vi "Bang-bang.vi"(1 "Feedback":dbl, 2 "Target":dbl, 3 "Tolerance":dbl, 4 "Slow point":dbl, 5 "Low Speed":dbl, 6 "High Speed":dbl) -> (0 "Out speed":dbl)   [LabVIEW 2015]
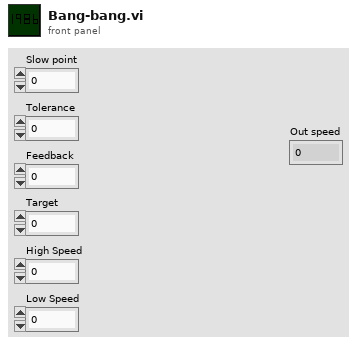
[diagram p1: front panel]
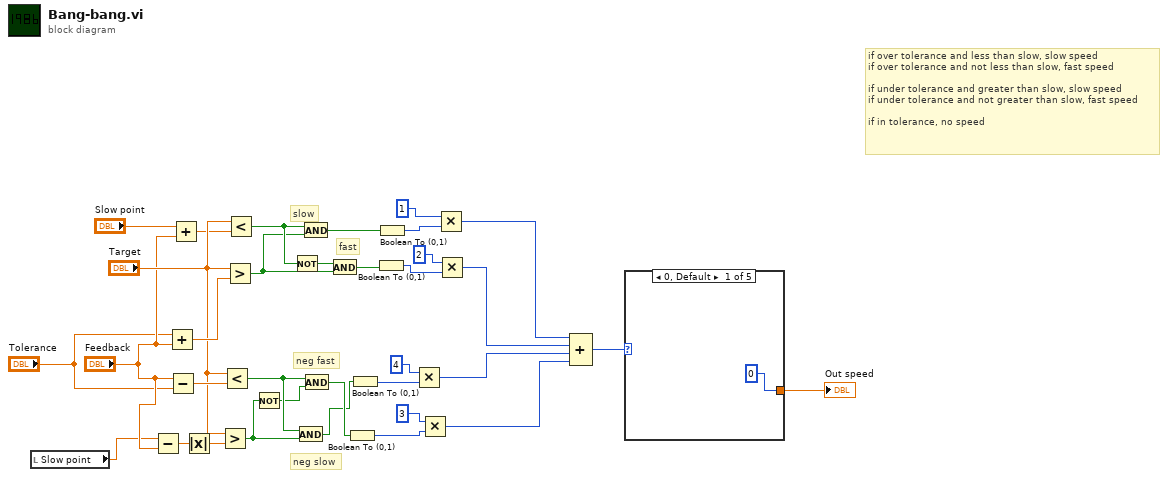
[diagram p0: block diagram]
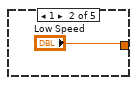
[diagram p2: hidden frame]
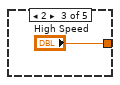
[diagram p3: hidden frame]
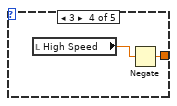
[diagram p4: hidden frame]
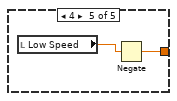
[diagram p5: hidden frame]
diagram:
  # "fast"
  # "neg fast"
  # "neg slow"
  # "slow"
  # "if over tolerance and less than slow, slow speed\nif over tolerance and not less than slow, fast speed\n\nif under tolerance and greater than slow, slow speed\nif under tolerance and not greater than slow, fast speed\n\nif in tolerance, no speed"
  n1 = local read "Slow point"() -> (w28:dbl)
  n2 = Subtract(x=w28, y="Feedback") -> (x-y=w2:dbl)
  n3 = Add(x="Tolerance", y="Feedback") -> (x+y=w34:dbl)
  n4 = Subtract(x="Feedback", y="Tolerance") -> (x-y=w33:dbl)
  n5 = Add(x="Slow point", y="Feedback") -> (x+y=w31:dbl)
  n6 = Absolute Value(x=w2) -> (abs(x)=w1:dbl)
  n7 = Greater?(x="Target", y=w1) -> (0:w22:bool)
  n8 = Less?(x="Target", y=w33) -> (x < y?=w24:bool)
  n9 = Greater?(x="Target", y=w34) -> (0:w25:bool)
  n10 = Less?(x="Target", y=w31) -> (x < y?=w26:bool)
  n11 = Not(x=w22) -> (.not. x?=w23:bool)
  n12 = Not(x=w26) -> (.not. x?=w27:bool)
  n13 = And(x=w24, y=w22) -> (x .and. y?=w3:bool)
  n14 = And(x=w26, y=w25) -> (x .and. y?=w20:bool)
  n15 = And(x=w24, y=w23) -> (x .and. y?=w4:bool)
  n16 = And(x=w27, y=w25) -> (x .and. y?=w21:bool)
  n17 = Boolean To (0,1)(Boolean=w4) -> (0, 1=w12:i16)
  n18 = Boolean To (0,1)(Boolean=w3) -> (0, 1=w14:i16)
  n19 = Boolean To (0,1)(Boolean=w21) -> (0, 1=w16:i16)
  n20 = Boolean To (0,1)(Boolean=w20) -> (0, 1=w19:i16)
  n21 = Multiply(x=i16 4, y=w14) -> (x*y=w10:i16)
  n22 = Multiply(x=i16 3, y=w12) -> (x*y=w11:i16)
  n23 = Multiply(x=i16 1, y=w19) -> (x*y=w8:i16)
  n24 = Multiply(x=i16 2, y=w16) -> (x*y=w9:i16)
  n25 = Compound Arithmetic op=ADD(w8, w9, w10, w11) -> (w7:i16)
  n26 = case shown="0, Default" w7 {
    tunnel: [0 "Low Speed" "High Speed" w39 w41] -> w6
    frame 0, Default {
    }
    frame 1 {
    }
    frame 2 {
    }
    frame 3 {
      n27 = local read "High Speed"() -> (w38:dbl)
      n28 = Negate(x=w38) -> (-x=w39:dbl)
    }
    frame 4 {
      n29 = local read "Low Speed"() -> (w40:dbl)
      n30 = Negate(x=w40) -> (-x=w41:dbl)
    }
  }
  "Out speed" <- w6
